vi "ServerRunCheck.vi"(0 "ROS in":T2={"topic port"=0, "Node"="", "topic"="", "type"="", "node port"=0, "error "={"status"=FALSE, "code"=0, "source"=""}, "Direction"=enum."Node", "APIs"=[], "Update (ms)"=1, "write queue"=1}) -> (1 "Running?":bool, 2 "ServerFound":T1={"vi name"="", "VI Refnum"=refnum, "queue"=refnum, "ROS"={"topic port"=0, "Node"="", "topic"="", "type"="", "node port"=0, "error "={"status"=FALSE, "code"=0, "source"=""}, "Direction"=enum."Node", "APIs"=[], "Update (ms)"=1, "write queue"=1}, "notifier"=refnum})   [LabVIEW 2012]
uses:
  <userlib>/ROSforLV/ROS/Code/SubVIs/_ROSControl.ctl
  <userlib>/ROSforLV/ROS/Code/SubVIs/_ROSDirection.ctl
  <userlib>/ROSforLV/ROS/Code/Console/Servers/ServerSubs/ServoInfo.ctl
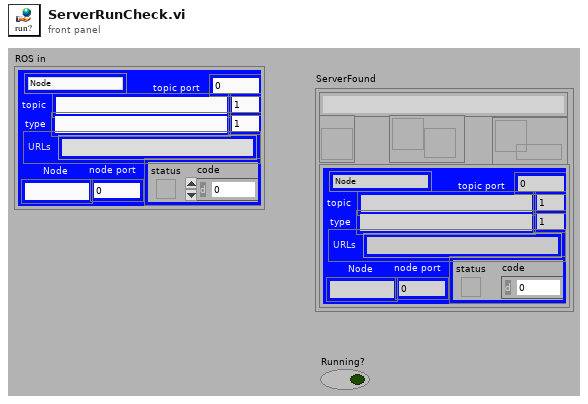
[diagram p1: front panel]
types:
  T1 = typedef "ServoInfo.ctl" = cluster{"vi name":string, "VI Refnum":refnum<vi>, "queue":refnum<queue>, "ROS":T2, "notifier":refnum<notifier>}
  T2 = typedef "_ROSControl.ctl" = cluster{"topic port":u16, "Node":string, "topic":string, "type":string, "node port":u16, "error ":errorcluster, "Direction":T3, "APIs":string[], "Update (ms)":u16, "write queue":u16}
  T3 = typedef "_ROSDirection.ctl" = enum16{"Node", "Publisher", "Subscriber", "Service Client"}
  T4 = enum16{"Add Server", "Clear Server", "Clear All", "Get Info"}
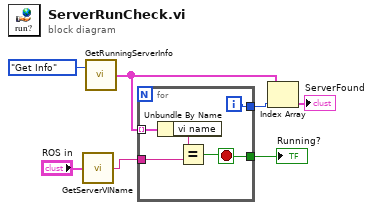
[diagram p0: block diagram]
diagram:
  n1 = call <userlib>:"GetServerVIName.vi"("ROS"="ROS in") -> ("vi name"=w2:string)
  n2 = call <userlib>:"GetRunningServerInfo.vi"("Task"=T4."Get Info") -> ("servers"=w4:T1[])  [unwired: 1 in, 2 out]
  n3 = for {
    tunnel: w4 -> [w12] mode=indexing
    tunnel: w2 -> [w10]
    tunnel: [w9] -> w3
    tunnel: [w8] -> w5
    i -> [w8]
    stop <- w9 stop-if-true
    n4 = Unbundle By Name(w12) -> ("vi name"=w11:string)
    n5 = Equal?(x=w11, y=w10) -> (x = y?=w9:bool)
  }
  "Running?" <- w3
  n6 = Index Array(array=w4, index=w5) -> (element=→"ServerFound":T1)
